vi "Navigate And Wait.vi"(0 "Display State In":T1, 1 "html Source (URL)":bool, 5 "Source":string, 7 "Timeout (Inf)":i32=-1, 9 "Container State":T2, 11 "error in (no error)":errorcluster) -> (4 "Display State Out":T1, 6 "Timed Out":bool, 15 "error out":errorcluster)   [LabVIEW 2020, in "WebView2 XControl.lvlib" / "WebView2 Control.xctl"]
uses:
  WebView2 Control.xctl
  <vilib>/_xctls/Container State.ctl
  State.ctl
  Webview2 Lib/WebView2 Control Object/WebView2 Control.lvclass
  <vilib>/_xctls/XControlSupport.lvlib
panel:
  # "Add Controls & Indicators that form the parameters of the method here. Hook them to the connector pane. Do not delete the controls & indicators that are already hooked to the connector pane.\n \nTo setup the parameters  for this method, right click on this item in the Project Tree & select \"Configure Method...\"."
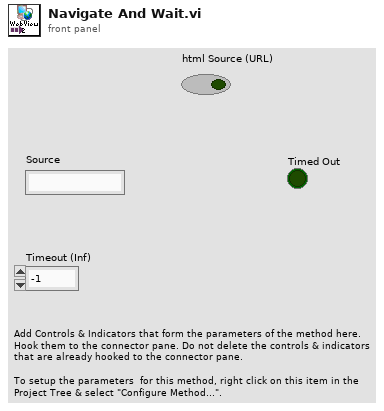
[diagram p1: front panel]
types:
  T1 = typedef "WebView2 XControl.lvlib/WebView2 Control.xctl/State.ctl" = cluster{"Control Object Ref":refnum<data-value>}
  T2 = typedef "XControlSupport.lvlib/Container State.ctl" = cluster{"Indicator?":bool, "Run Mode?":bool, " Refnum":refnum<vi>}
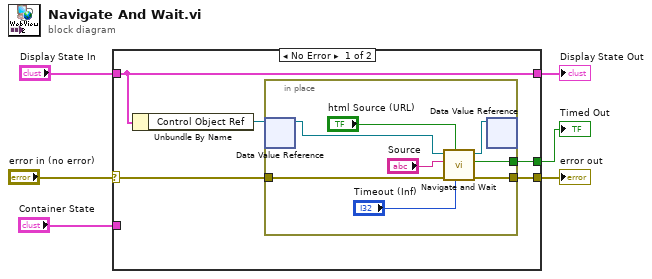
[diagram p0: block diagram]
diagram:
  n1 = case shown="No Error" "error in (no error)" {
    selector: "error in (no error)" -> [w10 w20]
    tunnel: "Display State In" -> [w7 w21]
    tunnel: "Container State" -> [_ _]
    tunnel: [w7 w21] -> w3
    tunnel: [w9 w20] -> w2
    tunnel: [w8 _] -> w1
    frame No Error {
      n2 = Unbundle By Name(w7) -> ("Control Object Ref"=w11:refnum<data-value>)
      n3 = in-place {
        in-place-border: w10 -> [w18]
        in-place-border: [w17] -> w9
        in-place-border: [w16] -> w8
        n4 = in-place-dvr #1(w11) -> (w19:refnum<class "WebView2 Control.lvclass">)  [unwired: 1 out]
        n5 = call "Navigate and Wait.vi"("Timeout (Inf)"="Timeout (Inf)", "html Source (URL)"="html Source (URL)", "error in (no error)"=w18, "Source"="Source", "WebView2 Control in"=w19) -> ("error out"=w17:errorcluster, "Timed Out"=w16:bool, "WebView2 Control out"=w12:refnum<class "WebView2 Control.lvclass">)  [unwired: 4 in]
        n6 = in-place-dvr #1(w12) -> ()  [unwired: 2 out]
      }
    }
    frame Error {
    }
  }
  "Display State Out" <- w3
  "error out" <- w2
  "Timed Out" <- w1
